vi "popularVideos.vi"(8 "error in (no error)":errorcluster, 11 "ThirdPartyYoutubeClass in":refnum<class "ThirdPartyYoutubeClass.lvclass">) -> (0 "error out":errorcluster, 2 "HashMap":T1, 3 "ThirdPartyYoutubeClass out":refnum<class "ThirdPartyYoutubeClass.lvclass">)   [LabVIEW 2018, in "ThirdPartyYoutubeClass.lvclass"]
uses:
  ThirdPartyYoutubeClass.lvclass
  Globals/HashMap.ctl
  Video Class/Video.lvclass
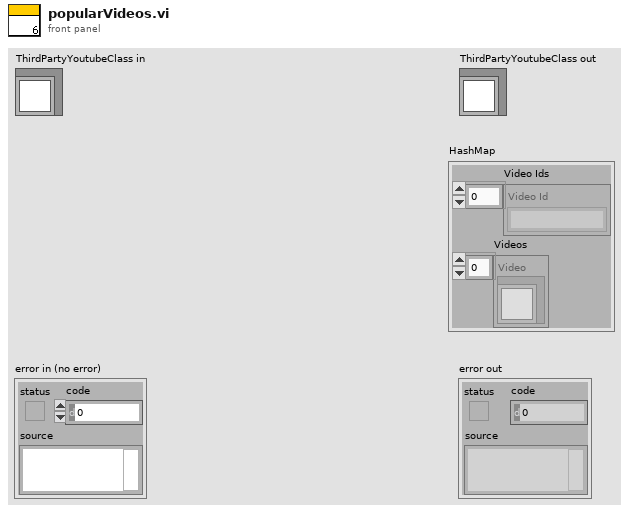
[diagram p1: front panel]
types:
  T1 = typedef "HashMap.ctl" = cluster{"Video Ids":string[], "Videos":refnum<class "Video.lvclass">[]}
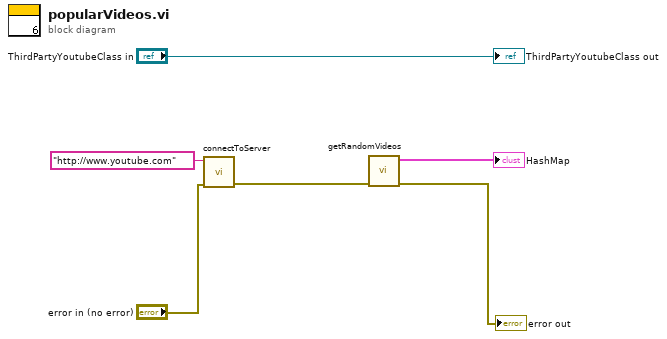
[diagram p0: block diagram]
diagram:
  n1 = call "connectToServer.vi"("error in (no error)"="error in (no error)", "server"="http://www.youtube.com") -> ("error out"=w3:errorcluster)  [unwired: 9 in]
  n2 = call "getRandomVideos.vi"("error in (no error)"=w3) -> ("error out"=→"error out":errorcluster, "HashMap"=→"HashMap":T1)  [unwired: 9 in]
  "ThirdPartyYoutubeClass out" <- "ThirdPartyYoutubeClass in"
